vi "Login.vi"(8 "error in (no error)":errorcluster) -> (0 "error out":errorcluster)   [LabVIEW 2017]
panel:
  in  "Close":bool
  in  "Cancel Button - Archive":bool
  in  "Username":string(combo)
  in  "Password":string
  in  "Login":bool
  # "User Login"
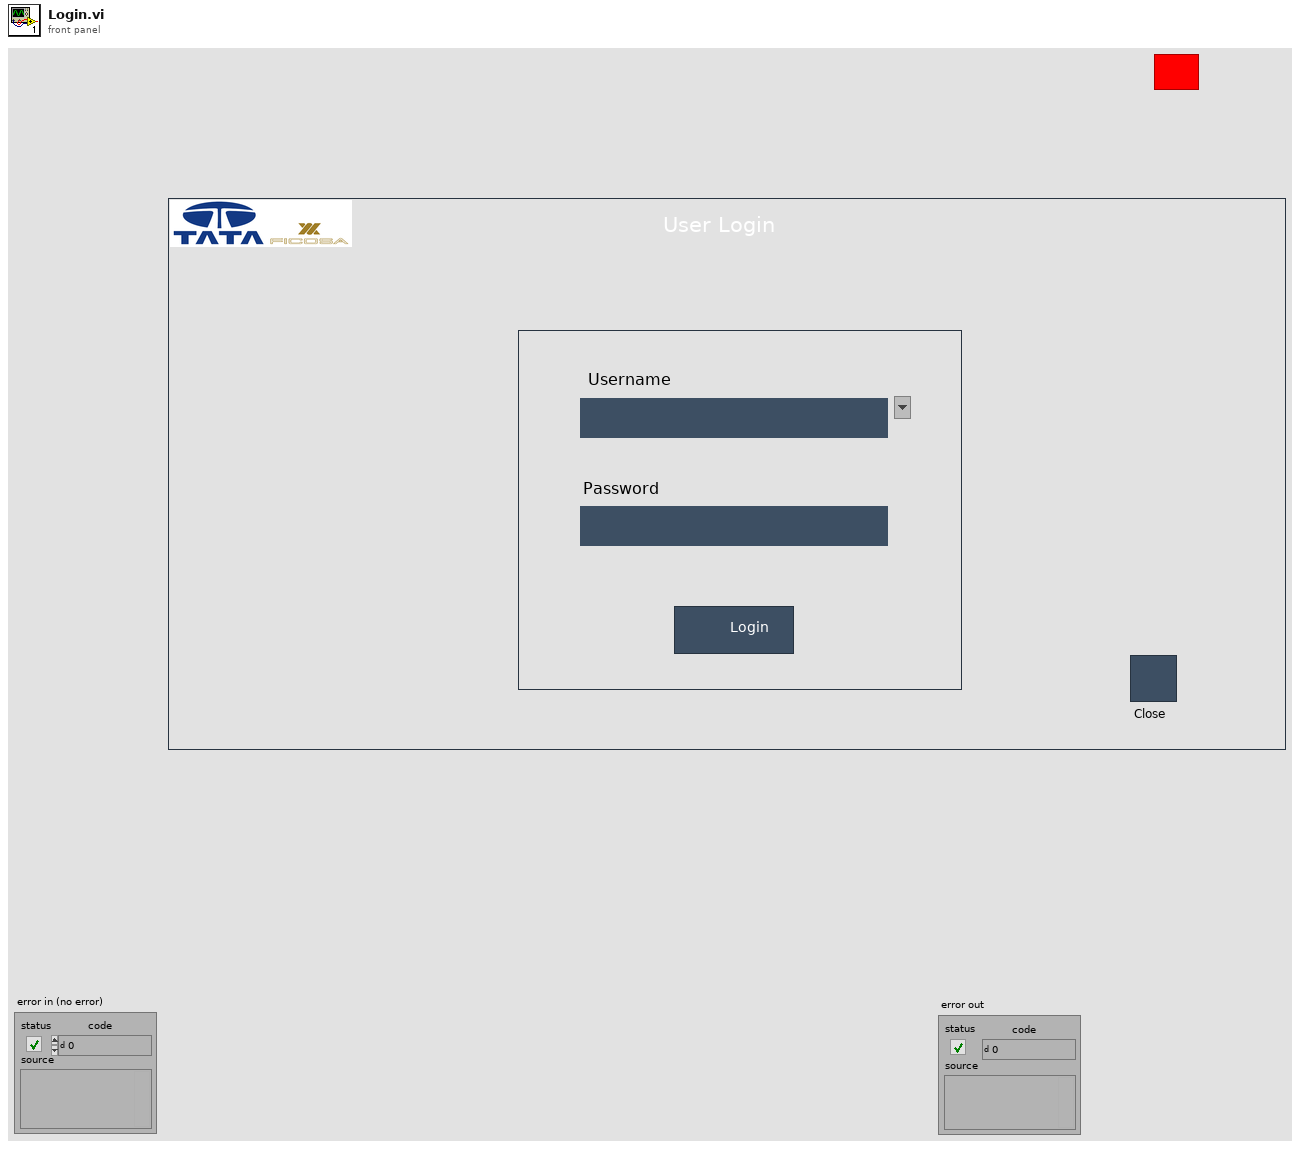
[diagram p1: front panel]
types:
  T1 = enum32{"invalid app kind", "Development System", "Run Time System", "Student Edition", "Embedded LabVIEW", "Evaluation", "Custom"}
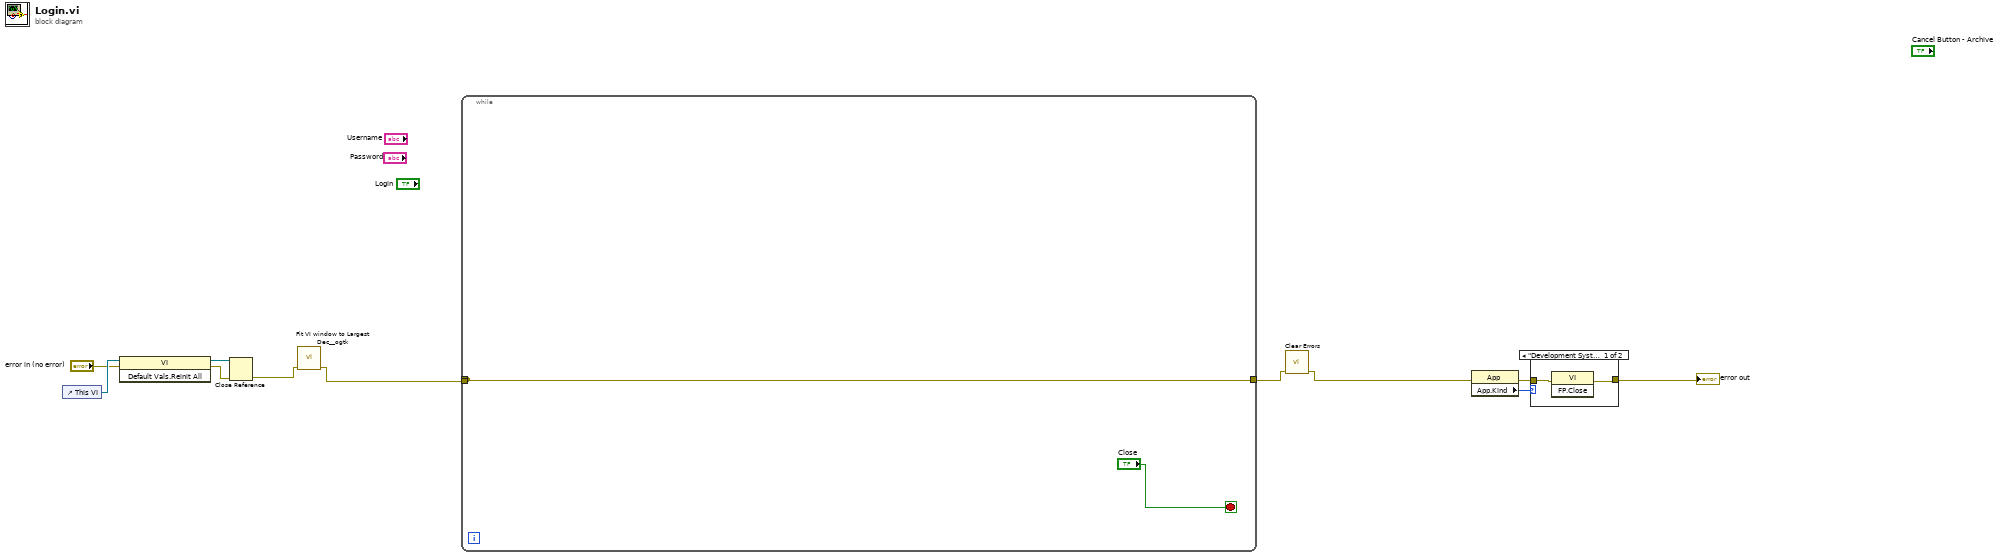
[diagram p0: block diagram]
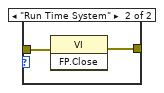
[diagram p2: hidden frame]
diagram:
  n1 = control-ref of="This VI"() -> (w11:refnum<vi>)
  n2 = invoke class="VI" method="Default Vals.Reinit All"(reference=w11, error in="error in (no error)") -> (reference out=w10:refnum<vi>, error out=w9:errorcluster)  [unwired: 1 in, 1 out]
  n3 = Close Reference(reference=w10, error in (no error)=w9) -> (error out=w2:errorcluster)
  n4 = call <userlib>:"Fit VI window to Largest Dec__ogtk.vi"("error in (no error)"=w2) -> ("error out"=w1:errorcluster)  [unwired: 5 in, 1 out]
  n5 = while {
    tunnel: [w13] -> _
    tunnel: [w13] -> w4
    tunnel: w1 -> [w13]
    stop <- "Close" stop-if-true
  }
  n6 = call <vilib>:"Clear Errors.vi"("error in (no error)"=w4) -> ("error out"=w3:errorcluster)  [unwired: 5 in, 1 out]
  n7 = property class="App"(error in=w3) -> (error out=w8:errorcluster, "App.Kind"=w7:T1)  [unwired: 1 in, 1 out]
  n8 = case shown="\"Development System\", Default" w7 {
    tunnel: w8 -> [w15 w17]
    tunnel: [w14 w16] -> w6
    frame "Development System", Default {
      n9 = invoke class="VI" method="FP.Close"(error in=w15) -> (error out=w14:errorcluster)  [unwired: 2 in, 2 out]
    }
    frame "Run Time System" {
      n10 = invoke class="VI" method="FP.Close"(error in=w17) -> (error out=w16:errorcluster)  [unwired: 2 in, 2 out]
    }
  }
  "error out" <- w6
